vi "DB Get Station Type.vi"(8 "error in (no error)":errorcluster) -> (0 "error out":errorcluster, 2 "Station Types":string[](array[string]))   [LabVIEW 2019, in "Control Experiment.lvclass"]
uses:
  Control Experiment.lvclass
  <vilib>/JDP Science/PostgreSQL Library/Connection/Execute Command (1D string results).vi
  <vilib>/JDP Science/PostgreSQL Library/Connection/Execute Command (Result).vi
  <vilib>/JDP Science/PostgreSQL Library/Result/Get all results as 1D strings array.vi
  <vilib>/JDP Science/PostgreSQL Library/Result/Get Column Headers.vi
  <vilib>/JDP Science/PostgreSQL Library/Result/Clear.vi
  <vilib>/JDP Science/PostgreSQL Library/Connection/PQ Connection.lvclass
  <userlib>/LevyLab/LV-Data/LV-Data.PG/PGPASS/PGPASS.lvlib
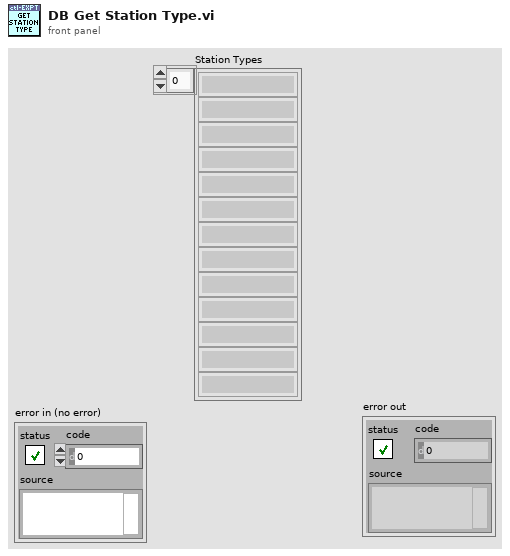
[diagram p1: front panel]
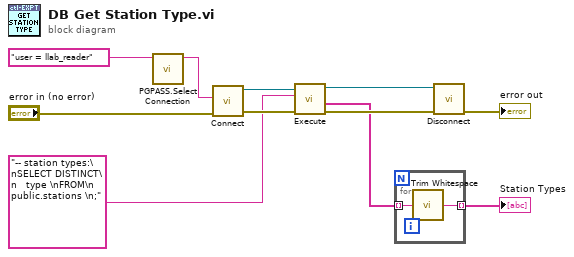
[diagram p0: block diagram]
diagram:
  n1 = call <userlib>:"PGPASS.Select Connection.vi"("search string"="user = llab_reader") -> ("connection string"=w11:string)  [unwired: 9 in, 1 out]
  n2 = call <vilib>:"Connect.vi"("error in (no error)"="error in (no error)", "Connection Strings"=w11) -> ("error out"=w9:errorcluster, "PQ Connection"=w10:refnum<class "PQ Connection.lvclass">)  [unwired: 8 in]
  n3 = call-poly <vilib>:"Execute.vi"("error in (no error)"=w9, "SQL"="-- station types:\nSELECT DISTINCT\n   type \nFROM\n   public.stations \n;" ("Address"), "PQ Connection in"=w10) -> ("error out"=w7:errorcluster, "Result (Rows or Columns)"=w1:string[], "PQ Connection out"=w8:refnum<class "PQ Connection.lvclass">)  [unwired: 4 in, 2 out]
  n4 = for {
    tunnel: w1 -> [w13] mode=indexing
    tunnel: [w12] -> w4 mode=indexing
    n5 = call <vilib>:"Trim Whitespace.vi"("string"=w13) -> ("trimmed string"=w12:string)  [unwired: 1 in]
  }
  "Station Types" <- w4
  n6 = call <vilib>:"Disconnect.vi"("error in (no error)"=w7, "PQ Connection in"=w8) -> ("error out"=→"error out":errorcluster)  [unwired: 9 in]
